vi "ABR-Append Data.vi"(0 "path":path, 9 "Array of levels tested":dbl[](array[numeric]), 11 "error in (no error)":errorcluster, 12 "Neural":dbl[][](array[numeric]), 13 "\"CM\"":dbl[][](array[numeric])) -> (15 "error out":errorcluster)   [LabVIEW 2020]
panel:
  out "path out":path
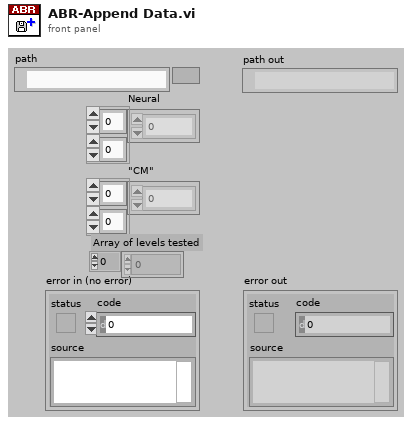
[diagram p1: front panel]
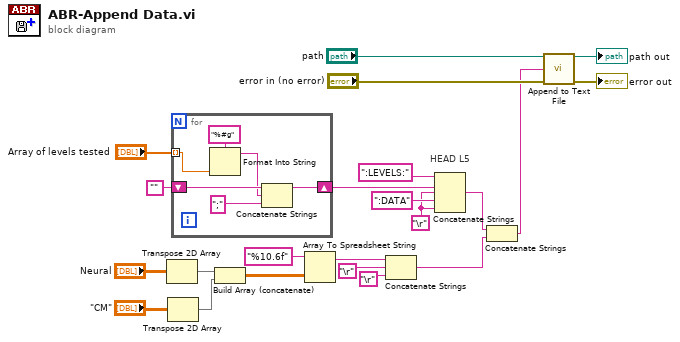
[diagram p0: block diagram]
diagram:
  w14 = "\r"
  # "HEAD L5"
  n1 = Transpose 2D Array(2D array="Neural") -> (transposed array=w4:dbl[][])
  n2 = Transpose 2D Array(2D array="\"CM\"") -> (transposed array=w3:dbl[][])
  n3 = for {
    shift-right: [w26] -> w15
    shift-left: "" -> [w28]
    tunnel: "Array of levels tested" -> [w25] mode=indexing
    n4 = Format Into String(format string="%#g", w25) -> (resulting string=w24:string)  [unwired: 2 in, 1 out]
    n5 = Concatenate Strings(w28, w24, ";") -> (w26:string)
  }
  n6 = Build Array (concatenate)(w4, w3) -> (w2:dbl[][])
  n7 = Array To Spreadsheet String(array=w2, 3:"%10.6f") -> (spreadsheet string=w10:string)  [unwired: 1 in]
  n8 = Concatenate Strings(w10, "\r", "\r") -> (w1:string)
  n9 = Concatenate Strings(":LEVELS:", w15, w14, ":DATA", w14) -> (w12:string)
  n10 = Concatenate Strings(w12, w1) -> (w7:string)
  n11 = call "Append to Text File.vi"("file path"="path", "text"=w7, "error in (no error)"="error in (no error)") -> ("file path out"=→"path out":path, "error out"=→"error out":errorcluster)  [unwired: 11 in]
